vi "initTable.vi"(8 "error in":errorcluster, 10 "Column Header Strings[]":string[](array[string]), 11 "Tbl Refnum in":refnum<vi>) -> (0 "error out":errorcluster, 3 "Tbl Refnum out":refnum<vi>)   [LabVIEW 2010]
uses:
  <vilib>/Utility/miscctls.llb/LVRowAndColumnTypeDef.ctl
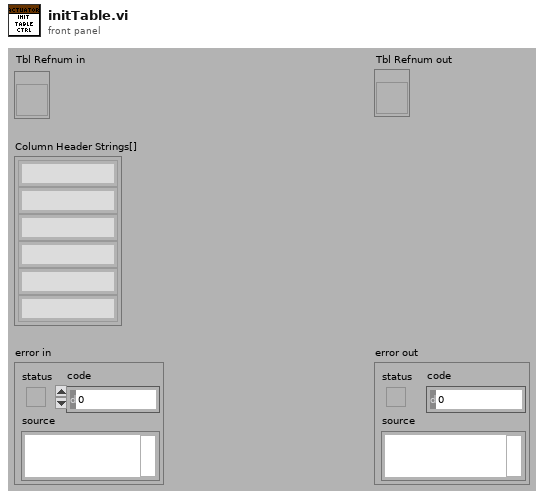
[diagram p1: front panel]
types:
  T1 = typedef "LVRowAndColumnTypeDef.ctl" = cluster{"Row":i32, "Column":i32}
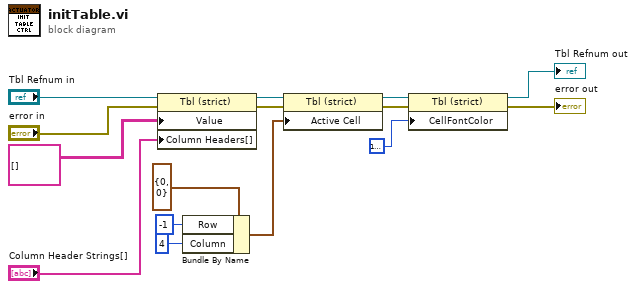
[diagram p0: block diagram]
diagram:
  n1 = property class="Tbl (strict)"(reference="Tbl Refnum in", error in="error in", "Value"=string[][] [], "Column Headers[]"="Column Header Strings[]") -> (reference out=w12:refnum<vi>, error out=w11:errorcluster)
  n2 = Bundle By Name(cluster=T1 {"Row"=0, "Column"=0} ("Active Cell:Active Cell"), "Row"=-1, "Column"=4) -> (w7:T1)
  n3 = property on="Property Node" class="Tbl (strict)"(reference=w12, error in=w11, "Active Cell"=w7) -> (reference out=w6:refnum<vi>, error out=w5:errorcluster)
  n4 = property on="Property Node" class="Tbl (strict)"(reference=w6, error in=w5, "CellFontColor"=u32 16777222) -> (reference out=→"Tbl Refnum out":refnum<vi>, error out=→"error out":errorcluster)
